vi "VISP Copy VI to Clipboard.vi"(8 "error in (no error)":errorcluster, 10 "Selected GObjects Only? (F)":bool, 11 "VI Refnum in":refnum<vi>) -> (0 "error out":errorcluster, 3 "dup VI Refnum":refnum<vi>)   [LabVIEW 2019, in "VI Snippet.lvlib"]
doc: "Copies the <b>VI Refnum in</b> block diagram content to the clipboard. If <b>Selected GObjects Only?</b> is True, this only copies the currently selected GObjects on the block diagram. Otherwise, all diagram content is copied.\n\nCreated by: Ryan Pacini"
uses:
  VI Snippet.lvlib
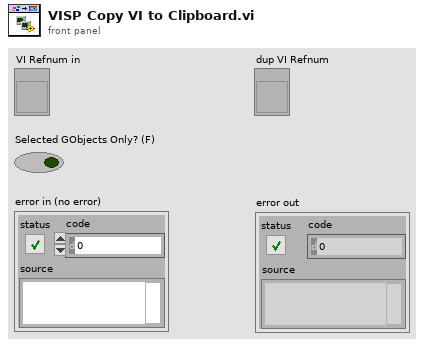
[diagram p1: front panel]
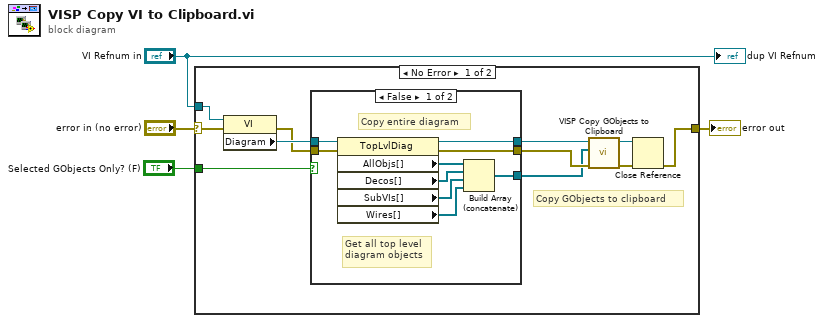
[diagram p0: block diagram]
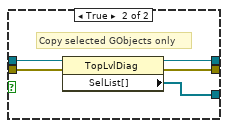
[diagram p2: hidden frame]
diagram:
  n1 = case shown="No Error" "error in (no error)" {
    selector: "error in (no error)" -> [w8 w30]
    tunnel: "VI Refnum in" -> [w7 _]
    tunnel: [w6 w30] -> w3
    tunnel: "Selected GObjects Only? (F)" -> [w5 _]
    frame No Error {
      # "Copy GObjects to clipboard"
      n2 = property class="VI"(reference=w7, error in=w8) -> (error out=w12:errorcluster, "Diagram"=w14:refnum<vi>)  [unwired: 1 out]
      n3 = case shown="False" w5 {
        tunnel: w14 -> [w24 w27]
        tunnel: [w23 w25] -> w13
        tunnel: w12 -> [w22 w29]
        tunnel: [w21 w28] -> w11
        tunnel: [w16 w26] -> w10
        frame False {
          # "Copy entire diagram"
          # "Get all top level\ndiagram objects"
          n4 = property class="TopLvlDiag"(reference=w24, error in=w22) -> (reference out=w23:refnum<vi>, error out=w21:errorcluster, "AllObjs[]"=w20:refnum<vi>[], "Decos[]"=w19:refnum<vi>[], "SubVIs[]"=w18:refnum<vi>[], "Wires[]"=w17:refnum<vi>[])
          n5 = Build Array (concatenate)(w20, w19, w18, w17) -> (w16:refnum<vi>[])
        }
        frame True {
          # "Copy selected GObjects only"
          n6 = property class="TopLvlDiag"(reference=w27, error in=w29) -> (reference out=w25:refnum<vi>, error out=w28:errorcluster, "SelList[]"=w26:refnum<vi>[])
        }
      }
      n7 = call "VISP Copy GObjects to Clipboard.vi"("error in (no error)"=w11, "GObjects"=w10, "Diagram in"=w13) -> ("error out"=w15:errorcluster, "Diagram out"=w9:refnum<vi>)  [unwired: 7 in]
      n8 = Close Reference(reference=w9, error in (no error)=w15) -> (error out=w6:errorcluster)
    }
    frame Error {
    }
  }
  "error out" <- w3
  "dup VI Refnum" <- "VI Refnum in"
